vi "gu_is_text_utf8.vi"(8 "error in":errorcluster, 11 "Encoded String":T1) -> (0 "error out":errorcluster, 3 "UTF-8":bool)   [LabVIEW 2020, in "G-Unicode.lvlib"]
uses:
  G-Unicode.lvlib
  Types/Encoded UTF-8 String.ctl
  lib/g_unicode_32.dll
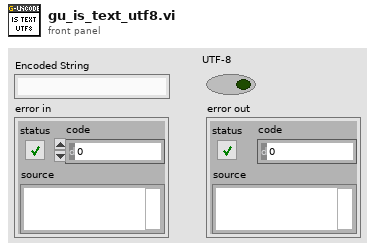
[diagram p1: front panel]
types:
  T1 = typedef "G-Unicode.lvlib/Encoded UTF-8 String.ctl" = string
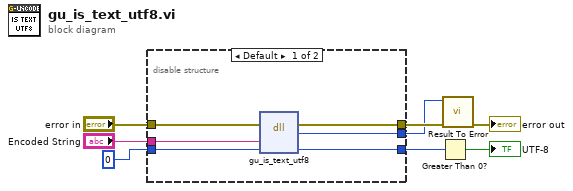
[diagram p0: block diagram]
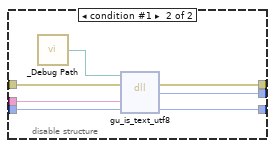
[diagram p2: hidden frame]
diagram:
  n1 = disable-structure shown="Default" {
    disable-tunnel: "Encoded String" -> [w12 w19]
    disable-tunnel: [w10 w17] -> w7
    disable-tunnel: "error in" -> [w14 w21]
    disable-tunnel: [w13 w20] -> w3
    disable-tunnel: 0 ("utf8") -> [w11 w16]
    disable-tunnel: [w9 w15] -> w1
    frame condition #0 (active) {
      n2 = dll-call lib="C:/github/dataflowg/g-unicode/src/LabVIEW/G-Unicode/lib/g_unicode_*.*" fn="gu_is_text_utf8"(error in=w14, "str"=w12, "is_utf8"=w11) -> (error out=w13:errorcluster, "result"=w9:i32, "is_utf8"=w10:i32)  [unwired: 3 in, 1 out]
    }
    frame condition #1 {
      n3 = call "_Debug Path.vi"() -> ("Debug Path"=w18:path)
      n4 = dll-call lib="?" fn="gu_is_text_utf8"(path in=w18, error in=w21, "str"=w19, "is_utf8"=w16) -> (error out=w20:errorcluster, "result"=w15:i32, "is_utf8"=w17:i32)  [unwired: 2 in, 1 out]
    }
  }
  n5 = Greater Than 0?(x=w7) -> (x > 0?=→"UTF-8":bool)
  n6 = call "Result To Error.vi"("error in (no error)"=w3, "Result Code"=w1) -> ("error out"=→"error out":errorcluster)  [unwired: 9 in]
